vi "Destroy.vi"(8 "error in (no error)":errorcluster, 11 "AprilTagDetector":refnum<data-value>) -> (0 "error out":errorcluster)   [LabVIEW 2020, in "g_ar_toolkit.feature_detection.lvlib" / "AprilTagDetector.lvclass"]
uses:
  AprilTagDetector.lvclass
  AprilTagDetector.lvclass/AprilTagDetector.ctl
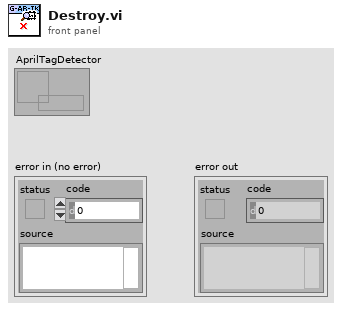
[diagram p1: front panel]
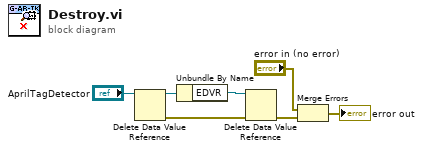
[diagram p0: block diagram]
diagram:
  n1 = Delete Data Value Reference(data value reference="AprilTagDetector") -> (data value=w6:refnum<class "AprilTagDetector.lvclass">, error out=w4:errorcluster)  [unwired: 1 in]
  n2 = Unbundle By Name(w6) -> ("EDVR"=w5:refnum<data-value>)
  n3 = Delete Data Value Reference(data value reference=w5, error in=w4) -> (error out=w2:errorcluster)  [unwired: 1 out]
  n4 = Merge Errors("error in (no error)", w2) -> (→"error out":errorcluster)
